vi "Commands.vi"(5 "VolatusAPI":refnum<class "VolatusAPI.lvclass">, 6 "State Loop Data in":T2, 7 "State Control":T1, 11 "State in":refnum<class "State.lvclass">) -> (3 "State out":refnum<class "State.lvclass">, 4 "State Loop Data":T2)   [LabVIEW 2023, in "VolatusSeq.lvlib" / "State.lvclass"]
uses:
  State.lvclass
  State Control.ctl
  Sequence Time.ctl
  Variables/Variables.lvclass
  State Loop Data.ctl
  Iteration Actions/Iteration Actions.lvclass
  Command.ctl
  Volatus/MessageQ/MessageQ.lvclass
  Format String/Format String.lvclass
  VolatusSeqConfig/Command Type.ctl
  messages/CmdDigital/Data.ctl
  messages/CmdAnalog/Data.ctl
  Send Type.ctl
  lv-vecto/Vecto/Channel DBL/Channel DBL.lvclass
  Transition/Transition.lvclass
  VolatusSeqConfig/Debug Flags.ctl
  Volatus/VolatusAPI/VolatusAPI.lvclass
  Iteration Actions/Iteration Actions.lvclass/Iteration Actions.ctl
  Volatus/MessageQ/MessageQ.lvclass/MessageQ.ctl
  lv-cdm/CDM-Config/ISO8601 Config.ctl
  lv-cdm/CDM-Config/Format.ctl
  lv-cdm/CDM-Config/Precision.ctl
  lv-cdm/CDM-Config/Timezone.ctl
  messages/StartLog/Data.ctl
  messages/StartLog/Class/Msg.lvclass/Msg.ctl
  Volatus/VolatusAPI/VolatusAPI.lvclass/VolatusAPI.ctl
  messages/StopLog/Data.ctl
  messages/StopLog/Class/Msg.lvclass/Msg.ctl
  Volatus/Event Level.ctl
  Variables/Variables.lvclass/Variables.ctl
  messages/CmdAnalog/Class/Msg.lvclass/Msg.ctl
  lv-vecto/Vecto/Channel DBL/Channel DBL.lvclass/Channel DBL.ctl
  messages/StartLog/Class/Msg.lvclass
  messages/StopLog/Class/Msg.lvclass
  messages/CmdAnalog/Class/Msg.lvclass
  lv-cdm/CDM-Config/ISO-8601 Format Strings.vi
  lv-vecto/Vecto/TCPMessageService/Send Message.vi
  <vilib>/Utility/error.llb/Error Cluster From Error Code.vi
  <vilib>/httpClient/POSTBuffer.vi
  lv-vecto/Vecto/Group DBL/Value by Index.vi
  lv-protoc/LV-Proto/Message/Message.lvclass
  State.lvclass/State.ctl
  lv-cdm/CDM-Config/CDM-Config.lvlib
  messages/StartLog/StartLog.lvlib
  messages/StopLog/StopLog.lvlib
  <vilib>/httpClient/LabVIEWHTTPClient.lvlib
  Volatus/Volatus.lvlib
  messages/CmdAnalogMultiple/Class/Msg.lvclass
  C:/dev/volatus/mts-volatus-super/libs/lv-volatus/messages/StartLog/Class/Msg.lvclass
  C:/dev/volatus/mts-volatus-super/libs/lv-protoc/LV-Proto/Message/Message.lvclass
  C:/dev/volatus/mts-volatus-super/libs/lv-volatus/messages/StopLog/Class/Msg.lvclass
  C:/dev/volatus/mts-volatus-super/libs/lv-volatus/messages/CmdAnalogMultiple/Class/Msg.lvclass
  VolatusSeq.lvlib
  VolatusSeqConfig/VolatusSeqConfig.lvlib
  messages/CmdDigital/CmdDigital.lvlib
  messages/CmdAnalog/CmdAnalog.lvlib
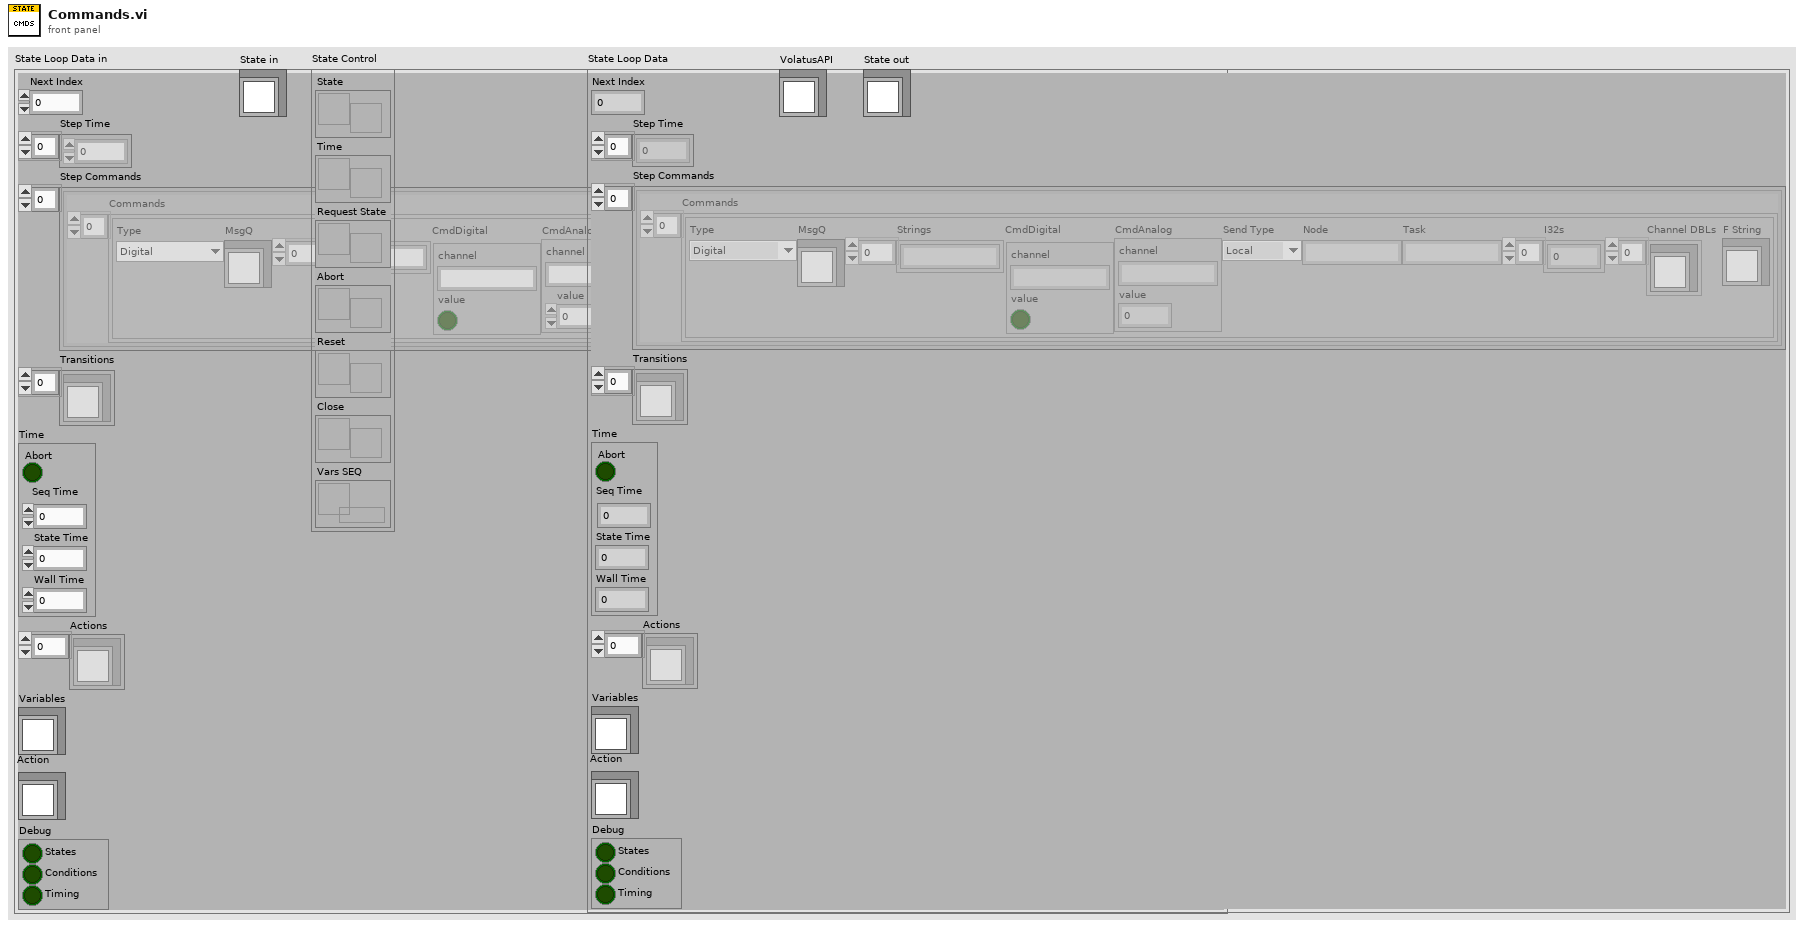
[diagram p1: front panel]
types:
  T1 = typedef "VolatusSeq.lvlib/State Control.ctl" = cluster{"State":refnum<notifier>, "Time":refnum<notifier>, "Request State":refnum<notifier>, "Abort":refnum<notifier>, "Reset":refnum<notifier>, "Close":refnum<notifier>, "Vars SEQ":refnum<queue>}
  T2 = typedef "VolatusSeq.lvlib/State.lvclass/State Loop Data.ctl" = cluster{"Next Index":i32, "Step Time":dbl[], "Step Commands":cluster{"Commands":T3[]}[], "Transitions":refnum<class "Transition.lvclass">[], "Time":T8, "Actions":refnum<class "Iteration Actions.lvclass">[], "Variables":refnum<class "Variables.lvclass">, "Action":refnum<class "Iteration Actions.lvclass">, "Debug":T9}
  T3 = typedef "VolatusSeq.lvlib/Command.ctl" = cluster{"Type":T4, "MsgQ":refnum<class "MessageQ.lvclass">, "Strings":string[], "CmdDigital":T5, "CmdAnalog":T6, "Send Type":T7, "Node":string, "Task":string, "I32s":i32[], "Channel DBLs":refnum<class "Channel DBL.lvclass">[], "F String":refnum<class "Format String.lvclass">}
  T4 = typedef "VolatusSeqConfig.lvlib/Command Type.ctl" = enum16{"Digital", "Numeric", "Transition", "Stop", "StartLog", "StopLog", "Start", "Event", "Error", "HTTP", "ResetVar", "IncVar", "DecVar", "SaveVar", "LoadVar", "AddVar", "SubVar", "SetVar", "AddToVar"}
  T5 = typedef "CmdDigital.lvlib/Data.ctl" = cluster{"channel":string, "value":bool}
  T6 = typedef "CmdAnalog.lvlib/Data.ctl" = cluster{"channel":string, "value":dbl}
  T7 = typedef "VolatusSeq.lvlib/Send Type.ctl" = enum16{"Local", "Remote"}
  T8 = typedef "VolatusSeq.lvlib/Sequence Time.ctl" = cluster{"Abort":bool, "Seq Time":dbl, "State Time":dbl, "Wall Time":dbl}
  T9 = typedef "VolatusSeqConfig.lvlib/Debug Flags.ctl" = cluster{"States":bool, "Conditions":bool, "Timing":bool}
  T10 = typedef "StartLog.lvlib/Data.ctl" = cluster{"series":string, "timestamp":string, "started_by":string, "groups":string[]}
  T11 = typedef "CDM-Config.lvlib/ISO8601 Config.ctl" = cluster{"Format":T12, "Precision":T13, "Timezone":T14}
  T12 = typedef "CDM-Config.lvlib/Format.ctl" = enum16{"Extended", "Basic"}
  T13 = typedef "CDM-Config.lvlib/Precision.ctl" = enum16{"Millisecond", "Second", "Minute", "Hour", "Day"}
  T14 = typedef "CDM-Config.lvlib/Timezone.ctl" = enum16{"UTC", "Local"}
  T15 = typedef "StopLog.lvlib/Data.ctl" = cluster{"reason":string, "groups":string[]}
  T16 = typedef "Volatus.lvlib/Event Level.ctl" = enum16{"Debug", "Info", "Warning", "Error"}
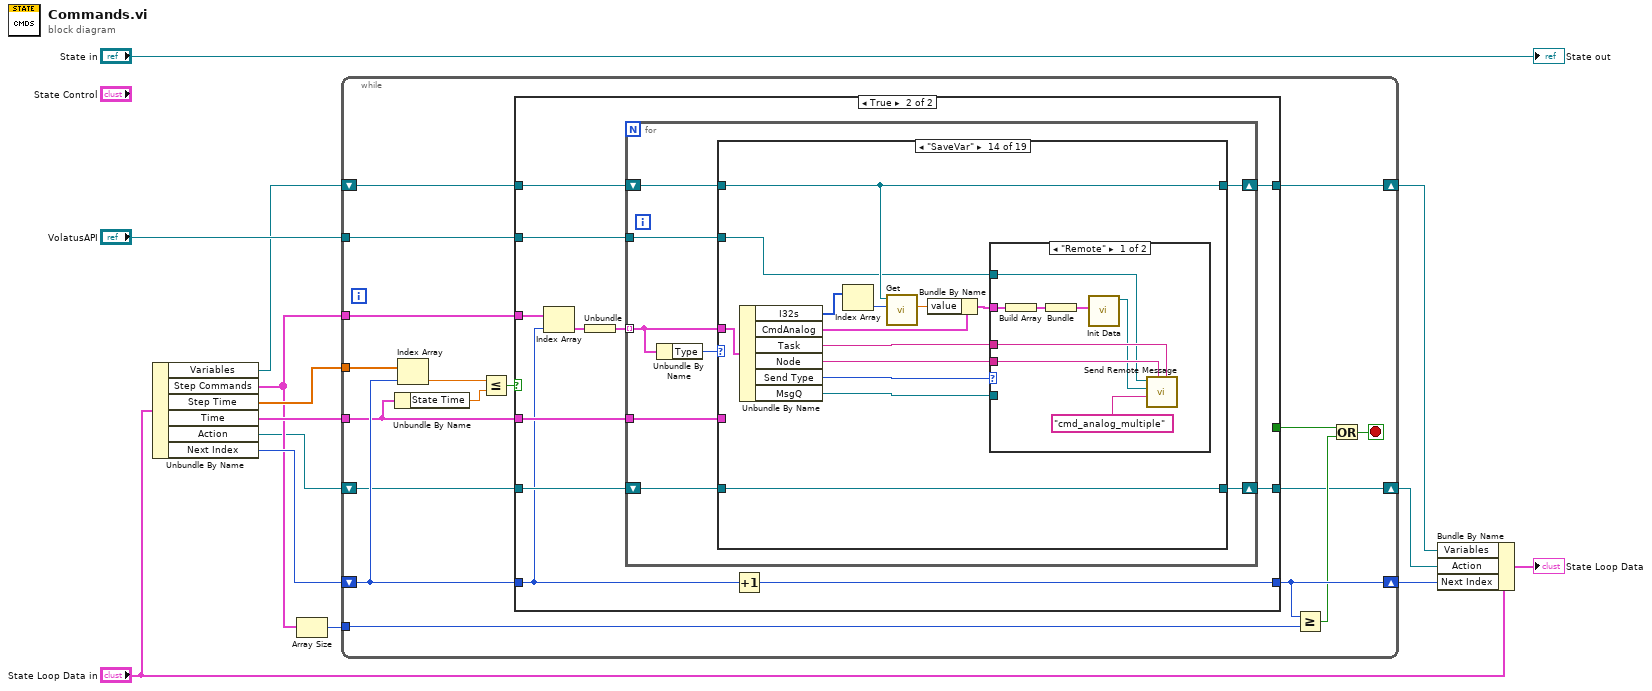
[diagram p0: block diagram]
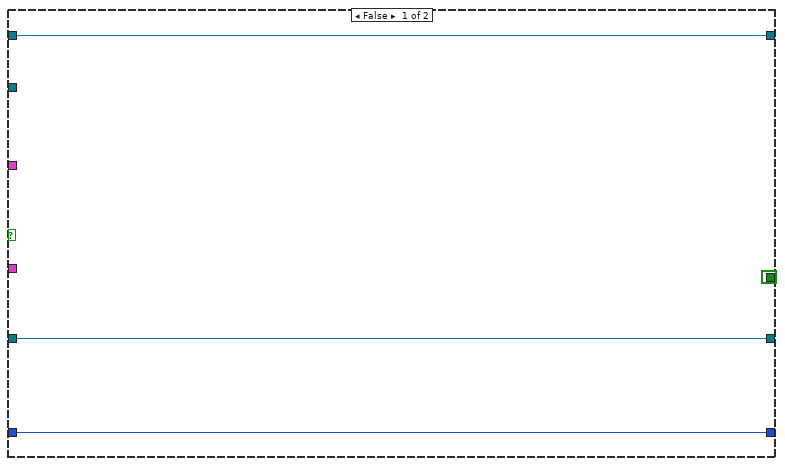
[diagram p2: hidden frame]
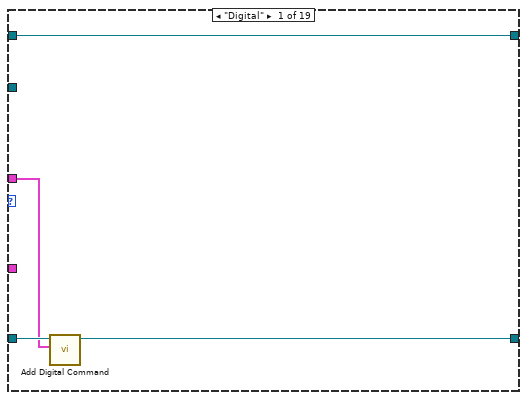
[diagram p3: hidden frame]
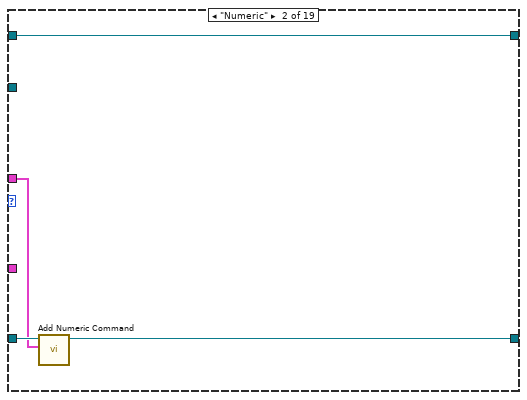
[diagram p4: hidden frame]
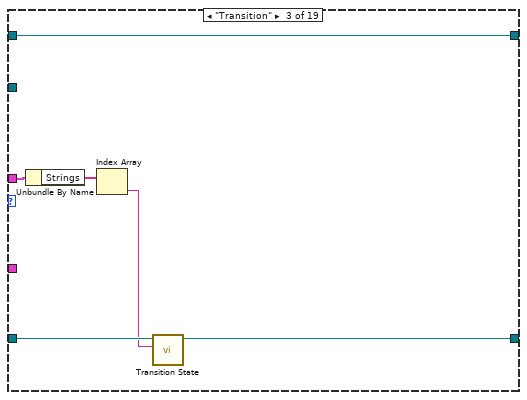
[diagram p5: hidden frame]
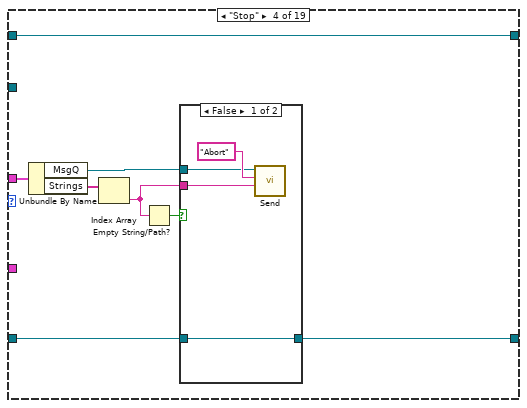
[diagram p6: hidden frame]
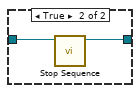
[diagram p7: hidden frame]
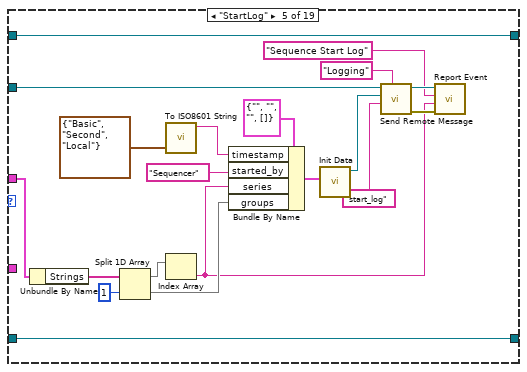
[diagram p8: hidden frame]
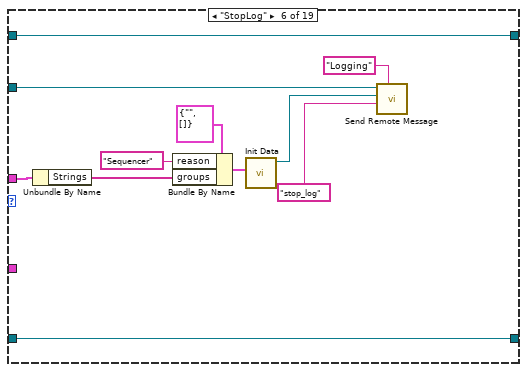
[diagram p9: hidden frame]
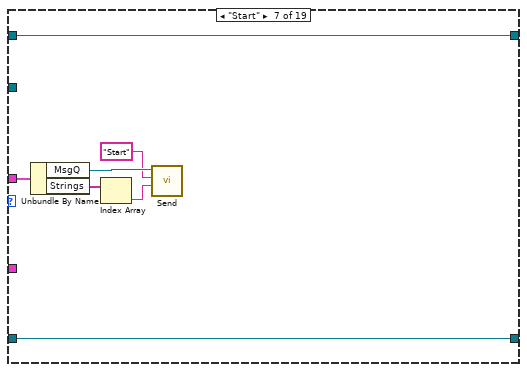
[diagram p10: hidden frame]
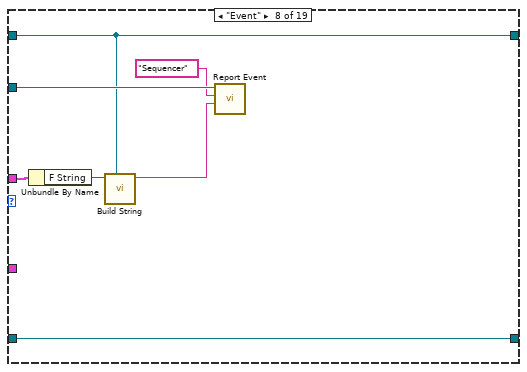
[diagram p11: hidden frame]
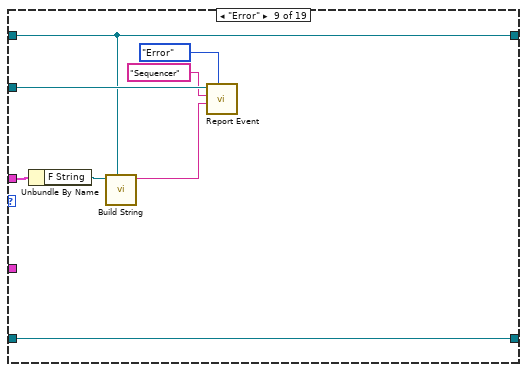
[diagram p12: hidden frame]
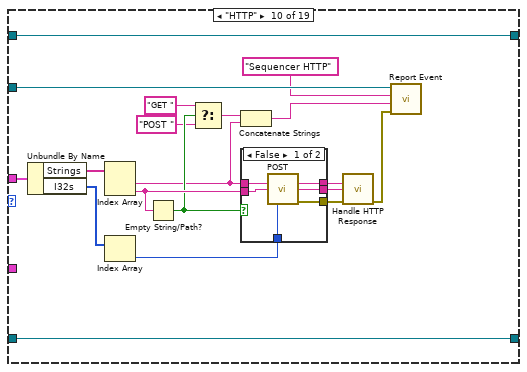
[diagram p13: hidden frame]
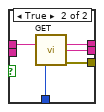
[diagram p14: hidden frame]
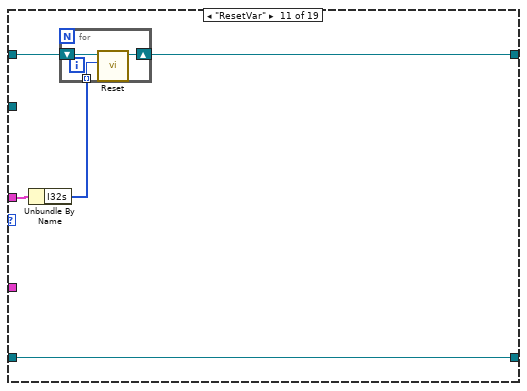
[diagram p15: hidden frame]
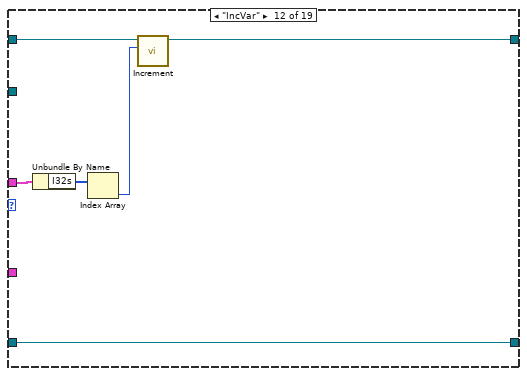
[diagram p16: hidden frame]
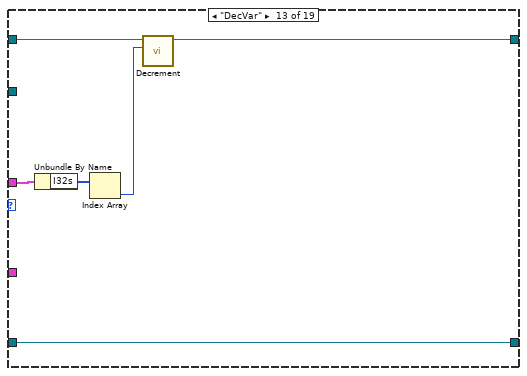
[diagram p17: hidden frame]
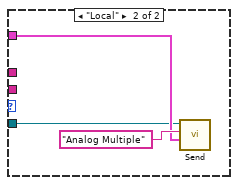
[diagram p18: hidden frame]
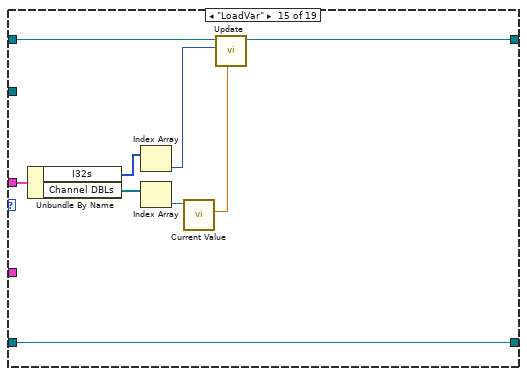
[diagram p19: hidden frame]
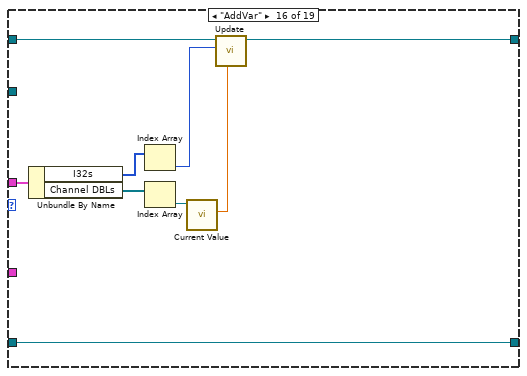
[diagram p20: hidden frame]
diagram:
  n1 = Unbundle By Name("State Loop Data in") -> ("Variables"=w4:refnum<class "Variables.lvclass">, "Step Commands"=w6:cluster{"Commands":T3[]}[], "Step Time"=w13:dbl[], "Time"=w8:T8, "Action"=w2:refnum<class "Iteration Actions.lvclass">, "Next Index"=w7:i32)
  n2 = Array Size(array=w6) -> (size(s)=w5:i32)
  n3 = while {
    tunnel: w13 -> [w31]
    tunnel: w8 -> [w23]
    shift-right: [w22] -> w10
    shift-left: w7 -> [w27]
    tunnel: w6 -> [w28]
    tunnel: "VolatusAPI" -> [w25]
    tunnel: w5 -> [w21]
    shift-right: [w17] -> w3
    shift-left: w4 -> [w18]
    shift-right: [w15] -> w1
    shift-left: w2 -> [w16]
    stop <- w20 stop-if-true
    n4 = Unbundle By Name(w23) -> ("State Time"=w24:dbl)
    n5 = Index Array(array=w31, index=w27) -> (element=w30:dbl)
    n6 = Less Or Equal?(x=w30, y=w24) -> (x <= y?=w29:bool)
    n7 = case shown="True" w29 {
      tunnel: w28 -> [_ w46]
      tunnel: w27 -> [w35 w36]
      tunnel: [w35 w41] -> w22
      tunnel: [TRUE _] -> w26
      tunnel: w25 -> [_ w43]
      tunnel: w23 -> [_ w42]
      tunnel: w18 -> [w33 w40]
      tunnel: [w33 w39] -> w17
      tunnel: w16 -> [w32 w38]
      tunnel: [w32 w37] -> w15
      frame False {
      }
      frame True {
        n8 = Index Array(array=w46, index=w36) -> (element=w45:cluster{"Commands":T3[]})
        n9 = Unbundle(w45) -> ("Commands"=w44:T3[])
        n10 = for {
          tunnel: w44 -> [w52] mode=indexing
          shift-right: [w50] -> w39
          shift-left: w40 -> [w51]
          tunnel: w43 -> [w49]
          tunnel: w42 -> [w54]
          shift-right: [w47] -> w37
          shift-left: w38 -> [w48]
          n11 = Unbundle By Name(w52) -> ("Type"=w53:T4)
          n12 = case shown="\"SaveVar\"" w53 {
            tunnel: w54 -> [_ _ _ _ _ _ _ _ _ _ _ _ _ _ _ _ _ _ _]
            tunnel: w52 -> [w55 w59 w65 w74 w89 w109 w119 w127 w135 w153 w168 w177 w182 w198 w217 w226 _ w235 w245]
            tunnel: w51 -> [w58 w62 w68 w76 w102 w113 w120 w123 w129 w154 w170 w179 w185 w195 w218 w227 w229 w236 w241]
            tunnel: [w58 w62 w68 w76 w102 w113 w120 w123 w129 w154 w169 w178 w184 w195 w216 w222 w229 w233 w238] -> w50
            tunnel: w49 -> [_ _ _ _ w96 w110 _ w126 w134 w149 _ _ _ w190 _ _ _ _ _]
            tunnel: w48 -> [w57 w61 w67 w73 w83 w103 w114 w121 w128 w150 w166 w174 w180 w186 w210 w219 w228 w230 w237]
            tunnel: [w56 w60 w66 w72 w83 w103 w114 w121 w128 w150 w166 w174 w180 w186 w210 w219 w228 w230 w237] -> w47
            frame "Digital" {
              n13 = call "Add Digital Command.vi"("Command"=w55, "Iteration Actions in"=w57) -> ("Iteration Actions out"=w56:refnum<class "Iteration Actions.lvclass">)  [unwired: 8 in, 1 out]
            }
            frame "Numeric" {
              n14 = call "Add Numeric Command.vi"("Command"=w59, "Iteration Actions in"=w61) -> ("Iteration Actions out"=w60:refnum<class "Iteration Actions.lvclass">)  [unwired: 8 in, 1 out]
            }
            frame "Transition" {
              n15 = Unbundle By Name(w65) -> ("Strings"=w64:string[])
              n16 = Index Array(array=w64) -> (element=w63:string)  [unwired: 1 in]
              n17 = call "Transition State.vi"("Next State"=w63, "Iteration Actions in"=w67) -> ("Iteration Actions out"=w66:refnum<class "Iteration Actions.lvclass">)  [unwired: 8 in, 1 out]
            }
            frame "Stop" {
              n18 = Unbundle By Name(w74) -> ("MsgQ"=w69:refnum<class "MessageQ.lvclass">, "Strings"=w75:string[])
              n19 = Index Array(array=w75) -> (element=w70:string)  [unwired: 1 in]
              n20 = Empty String/Path?(string/path=w70) -> (empty?=w71:bool)
              n21 = case shown="False" w71 {
                tunnel: w73 -> [w80 w82]
                tunnel: [w80 w81] -> w72
                tunnel: w70 -> [w79 _]
                tunnel: w69 -> [w77 _]
                frame False {
                  n22 = call "Send.vi"("Data"=w79, "ID"="Abort", "MessageQ in"=w77) -> ()  [unwired: 7 in, 2 out]
                }
                frame True {
                  n23 = call "Stop Sequence.vi"("Iteration Actions in"=w82) -> ("Iteration Actions out"=w81:refnum<class "Iteration Actions.lvclass">)  [unwired: 9 in, 1 out]
                }
              }
            }
            frame "StartLog" {
              n24 = Unbundle By Name(w89) -> ("Strings"=w88:string[])
              n25 = Split 1D Array(array=w88, index=1) -> (first subarray=w91:string[], second subarray=w90:string[])
              n26 = call "To ISO8601 String.vi"("Format Config"=T11 {"Format"=enum."Basic", "Precision"=enum."Second", "Timezone"=enum."Local"}) -> ("ISO 8601"=w99:string)  [unwired: 10 in]
              n27 = Index Array(array=w91) -> (element=w84:string)  [unwired: 1 in]
              n28 = Bundle By Name(cluster=T10 {"series"="", "timestamp"="", "started_by"="", "groups"=[]} ("Data"), "timestamp"=w99, "started_by"="Sequencer", "series"=w84, "groups"=w90) -> (w95:T10)
              n29 = call "Init Data.vi"("Data"=w95) -> ("Msg out"=w98:refnum<class "Msg.lvclass">)  [unwired: 10 in]
              n30 = call "Send Remote Message.vi"("Target Name"="Logging", "Message Type"="start_log", "Message"=w98, "VolatusAPI in"=w96) -> ("error out"=w86:errorcluster, "VolatusAPI out"=w87:refnum<class "VolatusAPI.lvclass">)  [unwired: 6 in]
              n31 = call "Report Event.vi"("error in (no error)"=w86, "Message"=w84, "Context"="Sequence Start Log" ("Target Name"), "VolatusAPI in"=w87) -> ()  [unwired: 6 in, 2 out]
            }
            frame "StopLog" {
              n32 = Unbundle By Name(w109) -> ("Strings"=w107:string[])
              n33 = Bundle By Name(cluster=T15 {"reason"="", "groups"=[]} ("StopLog"), "reason"="Sequencer", "groups"=w107) -> (w105:T15)
              n34 = call "Init Data.vi"("Data"=w105) -> ("Msg out"=w104:refnum<class "Msg.lvclass">)  [unwired: 10 in]
              n35 = call "Send Remote Message.vi"("Target Name"="Logging", "Message Type"="stop_log", "Message"=w104, "VolatusAPI in"=w110) -> ()  [unwired: 6 in, 2 out]
            }
            frame "Start" {
              n36 = Unbundle By Name(w119) -> ("MsgQ"=w117:refnum<class "MessageQ.lvclass">, "Strings"=w118:string[])
              n37 = Index Array(array=w118) -> (element=w115:string)  [unwired: 1 in]
              n38 = call "Send.vi"("Data"=w115, "ID"="Start", "MessageQ in"=w117) -> ()  [unwired: 7 in, 2 out]
            }
            frame "Event" {
              n39 = Unbundle By Name(w127) -> ("F String"=w124:refnum<class "Format String.lvclass">)
              n40 = call "Build String.vi"("Variables"=w123, "Format String in"=w124) -> ("String"=w122:string)  [unwired: 8 in, 1 out]
              n41 = call "Report Event.vi"("Message"=w122, "Context"="Sequencer", "VolatusAPI in"=w126) -> ()  [unwired: 7 in, 2 out]
            }
            frame "Error" {
              n42 = Unbundle By Name(w135) -> ("F String"=w131:refnum<class "Format String.lvclass">)
              n43 = call "Build String.vi"("Variables"=w129, "Format String in"=w131) -> ("String"=w130:string)  [unwired: 8 in, 1 out]
              n44 = call "Report Event.vi"("Level (Info)"=Event_Level."Error", "Message"=w130, "Context"="Sequencer", "VolatusAPI in"=w134) -> ()  [unwired: 6 in, 2 out]
            }
            frame "HTTP" {
              n45 = Unbundle By Name(w153) -> ("Strings"=w152:string[], "I32s"=w137:i32[])
              n46 = Index Array(array=w152) -> (element #1=w143:string, element #2=w151:string)  [unwired: 2 in]
              n47 = Index Array(array=w137) -> (element=w136:i32)  [unwired: 1 in]
              n48 = Empty String/Path?(string/path=w151) -> (empty?=w147:bool)
              n49 = Select(t="GET ", s=w147, f="POST ") -> (s? t:f=w144:string)
              n50 = Concatenate Strings(w144, w143) -> (w142:string)
              n51 = case shown="False" w147 {
                tunnel: w143 -> [w160 w165]
                tunnel: w151 -> [w159 _]
                tunnel: [w158 w164] -> w140
                tunnel: [w157 w163] -> w139
                tunnel: [w156 w162] -> w141
                tunnel: w136 -> [w155 w161]
                frame False {
                  n52 = call-poly <vilib>:"POST.vi"("url"=w160, "buffer"=w159, "timeout (10000)"=w155) -> ("headers"=w158:string, "body"=w157:string, "error out"=w156:errorcluster)  [unwired: 9 in, 1 out]
                }
                frame True {
                  n53 = call <vilib>:"GET.vi"("url"=w165, "timeout (10000)"=w161) -> ("headers"=w164:string, "body"=w163:string, "error out"=w162:errorcluster)  [unwired: 10 in, 1 out]
                }
              }
              n54 = call "Handle HTTP Response.vi"("Headers"=w140, "Body"=w139, "error in (no error)"=w141) -> ("error out"=w138:errorcluster)  [unwired: 12 in]
              n55 = call "Report Event.vi"("error in (no error)"=w138, "Message"=w142, "Context"="Sequencer HTTP", "VolatusAPI in"=w149) -> ()  [unwired: 6 in, 2 out]
            }
            frame "ResetVar" {
              n56 = Unbundle By Name(w168) -> ("I32s"=w167:i32[])
              n57 = for {
                shift-right: [w172] -> w169
                shift-left: w170 -> [w173]
                tunnel: w167 -> [w171] mode=indexing
                n58 = call "Reset.vi"("Index"=w171, "Variables in"=w173) -> ("Variables out"=w172:refnum<class "Variables.lvclass">)  [unwired: 9 in]
              }
            }
            frame "IncVar" {
              n59 = Unbundle By Name(w177) -> ("I32s"=w176:i32[])
              n60 = Index Array(array=w176) -> (element=w175:i32)  [unwired: 1 in]
              n61 = call "Increment.vi"("Index"=w175, "Variables in"=w179) -> ("Variables out"=w178:refnum<class "Variables.lvclass">)  [unwired: 7 in, 2 out]
            }
            frame "DecVar" {
              n62 = Unbundle By Name(w182) -> ("I32s"=w183:i32[])
              n63 = Index Array(array=w183) -> (element=w181:i32)  [unwired: 1 in]
              n64 = call "Decrement.vi"("Index"=w181, "Variables in"=w185) -> ("Variables out"=w184:refnum<class "Variables.lvclass">)  [unwired: 7 in, 2 out]
            }
            frame "SaveVar" {
              n65 = Unbundle By Name(w198) -> ("I32s"=w197:i32[], "CmdAnalog"=w194:T6, "Task"=w188:string, "Node"=w187:string, "Send Type"=w189:T7, "MsgQ"=w191:refnum<class "MessageQ.lvclass">)
              n66 = Index Array(array=w197) -> (element=w196:i32)  [unwired: 1 in]
              n67 = call <vilib>:"Get.vi"("Index"=w196, "Variables in"=w195) -> ("Value"=w193:dbl)  [unwired: 9 in]
              n68 = Bundle By Name(cluster=w194, "value"=w193) -> (w192:T6)
              n69 = case shown="\"Remote\"" w189 {
                tunnel: w192 -> [w201 w208]
                tunnel: w191 -> [_ w207]
                tunnel: w190 -> [w204 _]
                tunnel: w188 -> [w205 _]
                tunnel: w187 -> [w206 _]
                frame "Remote" {
                  n70 = Build Array(w201) -> (w200:T6[])
                  n71 = Bundle(w200) -> (w199:cluster{T6[]})  [unwired: 1 in]
                  n72 = call "Init Data.vi"("Data"=w199) -> ("Msg out"=w203:refnum<class "Msg.lvclass">)  [unwired: 10 in]
                  n73 = call "Send Remote Message.vi"("Target Task (None)"=w205, "Target Name"=w206, "Message Type"="cmd_analog_multiple", "Message"=w203, "VolatusAPI in"=w204) -> ()  [unwired: 5 in, 2 out]
                }
                frame "Local" {
                  n74 = call "Send.vi"("Data"=w208, "ID"="Analog Multiple", "MessageQ in"=w207) -> ()  [unwired: 7 in, 2 out]
                }
              }
            }
            frame "LoadVar" {
              n75 = Unbundle By Name(w217) -> ("I32s"=w215:i32[], "Channel DBLs"=w213:refnum<class "Channel DBL.lvclass">[])
              n76 = Index Array(array=w215) -> (element=w214:i32)  [unwired: 1 in]
              n77 = Index Array(array=w213) -> (element=w212:refnum<class "Channel DBL.lvclass">)  [unwired: 1 in]
              n78 = call "Current Value.vi"("Channel in"=w212) -> ("Scaled"=w211:dbl)  [unwired: 6 in, 4 out]
              n79 = call "Update.vi"("Value"=w211, "Index"=w214, "Variables in"=w218) -> ("Variables out"=w216:refnum<class "Variables.lvclass">)  [unwired: 8 in]
            }
            frame "AddVar" {
              n80 = Unbundle By Name(w226) -> ("I32s"=w225:i32[], "Channel DBLs"=w224:refnum<class "Channel DBL.lvclass">[])
              n81 = Index Array(array=w225) -> (element=w220:i32)  [unwired: 1 in]
              n82 = Index Array(array=w224) -> (element=w223:refnum<class "Channel DBL.lvclass">)  [unwired: 1 in]
              n83 = call "Current Value.vi"("Channel in"=w223) -> ("Scaled"=w221:dbl)  [unwired: 6 in, 4 out]
              n84 = call "Update.vi"("Value"=w221, "Index"=w220, "Variables in"=w227) -> ("Variables out"=w222:refnum<class "Variables.lvclass">)  [unwired: 8 in]
            }
            frame "SubVar" {
            }
            frame "SetVar" {
              n85 = Unbundle By Name(w235) -> ("I32s"=w234:i32[], "CmdAnalog.value"=w231:dbl)
              n86 = Index Array(array=w234) -> (element=w232:i32)  [unwired: 1 in]
              n87 = call "Update.vi"("Value"=w231, "Index"=w232, "Variables in"=w236) -> ("Variables out"=w233:refnum<class "Variables.lvclass">)  [unwired: 8 in]
            }
            frame "AddToVar" {
              n88 = Unbundle By Name(w245) -> ("I32s"=w244:i32[], "CmdAnalog.value"=w242:dbl)
              n89 = Index Array(array=w244) -> (element=w240:i32)  [unwired: 1 in]
              n90 = call <vilib>:"Get.vi"("Index"=w240, "Variables in"=w241) -> ("Value"=w243:dbl)  [unwired: 9 in]
              n91 = Add(x=w243, y=w242) -> (x+y=w239:dbl)
              n92 = call "Update.vi"("Value"=w239, "Index"=w240, "Variables in"=w241) -> ("Variables out"=w238:refnum<class "Variables.lvclass">)  [unwired: 8 in]
            }
          }
        }
        n93 = Increment(x=w36) -> (x+1=w41:i32)
      }
    }
    n94 = Greater Or Equal?(x=w22, y=w21) -> (x >= y?=w19:bool)
    n95 = Or(x=w26, y=w19) -> (x .or. y?=w20:bool)
  }
  n96 = Bundle By Name(cluster="State Loop Data in", "Variables"=w3, "Action"=w1, "Next Index"=w10) -> (→"State Loop Data":T2)
  "State out" <- "State in"
